vi "Exemple_Metrics_Mean_Poisson_Deviance.vi"() -> ()   [LabVIEW 2020]
uses:
  Objet/3 - Model selection and evaluation/3.3 - Metrics and scoring/mean_poisson_deviance/Mean_Poisson_Deviance.vi
panel:
  out "Score":string
  out "error out":errorcluster caption="sortie d'erreur"
  in  "mean_poisson_deviance":cluster{"sample_weight":dbl[]}
  in  "error in (no error)":errorcluster caption="entrée d'erreur (pas d'erreur)"
  in  "y_pred":string[][](array[string])=[["0,5"], ["0,5"], ["2"], ["2"]]
  in  "y_true":string[][](array[string])=[["2"], ["0"], ["1"], ["4"]]
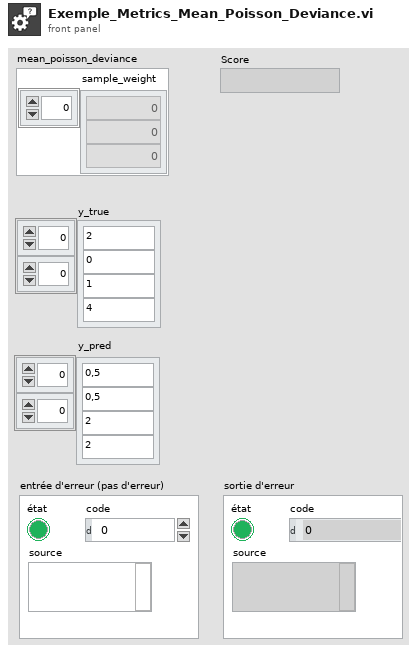
[diagram p1: front panel]
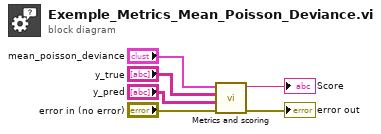
[diagram p0: block diagram]
diagram:
  n1 = call-poly "Metrics and scoring.vi"("error in (no error)"="error in (no error)", "y_pred"="y_pred", "y_true"="y_true", "mean_poisson_deviance"="mean_poisson_deviance") -> ("error out"=→"error out":errorcluster, "Score"=→"Score":string)  [unwired: 6 in]
